vi "Write_TDMS_v00.vi"(8 "error in":errorcluster, 9 "Waveform":waveform(dbl)[](array[waveform]) caption="wfm", 10 "File Name":path=path "C:/Documents and Settings/QIM/My Documents/LabVIEW Data/111016-discord-gain9-seed40-3/ele-0000mV-d0150mV-g9-s40.lvm", 11 "Record Data":bool) -> (0 "error out":errorcluster)   [LabVIEW 2011]
panel:
  out "Filename Out":path
  out "Saving Data":bool
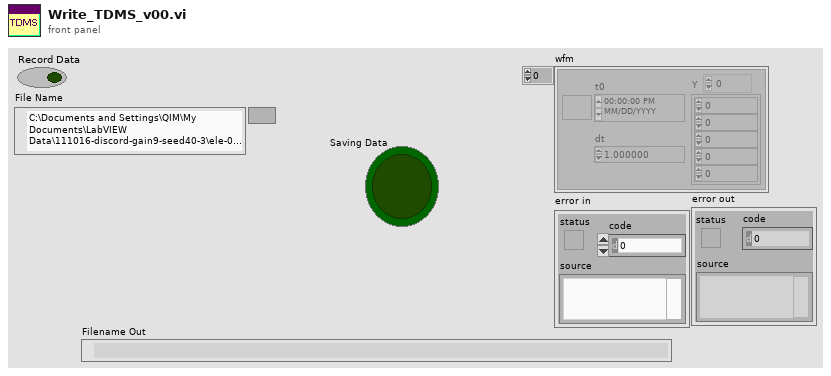
[diagram p1: front panel]
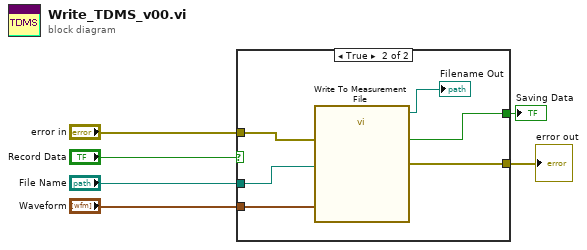
[diagram p0: block diagram]
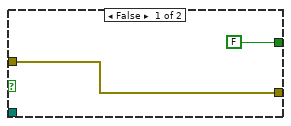
[diagram p2: hidden frame]
diagram:
  n1 = case shown="True" "Record Data" {
    tunnel: "Waveform" -> [_ w14]
    tunnel: "error in" -> [w8 w13]
    tunnel: "File Name" -> [_ w12]
    tunnel: [w8 w11] -> w2
    tunnel: [FALSE ("Saving Data") w10] -> w1
    frame False {
    }
    frame True {
      n2 = call "Write To Measurement File"("Signals"=w14, "error in (no error)"=w13, "Filename"=w12) -> ("Filename Out"=→"Filename Out":path, "Saving Data"=w10:bool, "error out"=w11:errorcluster)  [unwired: 14 in]
    }
  }
  "error out" <- w2
  "Saving Data" <- w1
